vi "overwrite.vi"(0 "Enable":bool=TRUE, 4 "Overwrite":path=path "C:/Users/Clavius/Desktop/Database Query files/New_Database_Query.hdf5" caption="Overwrite path", 5 "error in (no error)":errorcluster) -> (14 "Save folder":path=path "C:/Users/Clavius/Desktop/Database Query files/New_Database_Query.hdf5" caption="File path", 17 "Cancelled?":bool, 18 "Overwrite exsisting file":bool, 19 "error out":errorcluster)   [LabVIEW 2012]
doc: "Displays a standard dialog box that prompts users to enter information, such as a user name and password.\n--------------------\n\nThis Express VI is configured as follows:\n\nMessage to Display to the User:A file with the name you have specificied already exsists. \nThe inputs are:"
panel:
  in  "OK2 2":bool caption="OK2"
  in  "New Save folder":path caption="Change Name:"
  out "String":string="A file with the name you have specificied already exsists. "
  in  "OK2":bool
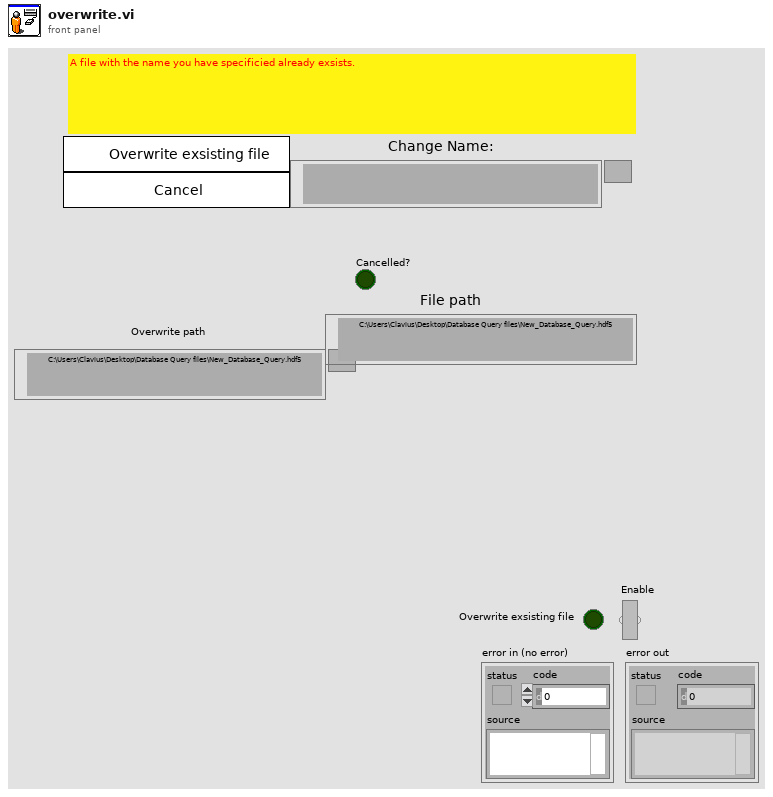
[diagram p1: front panel]
types:
  T1 = cluster{"Input Name":string, "Input Data Type":i32}[]
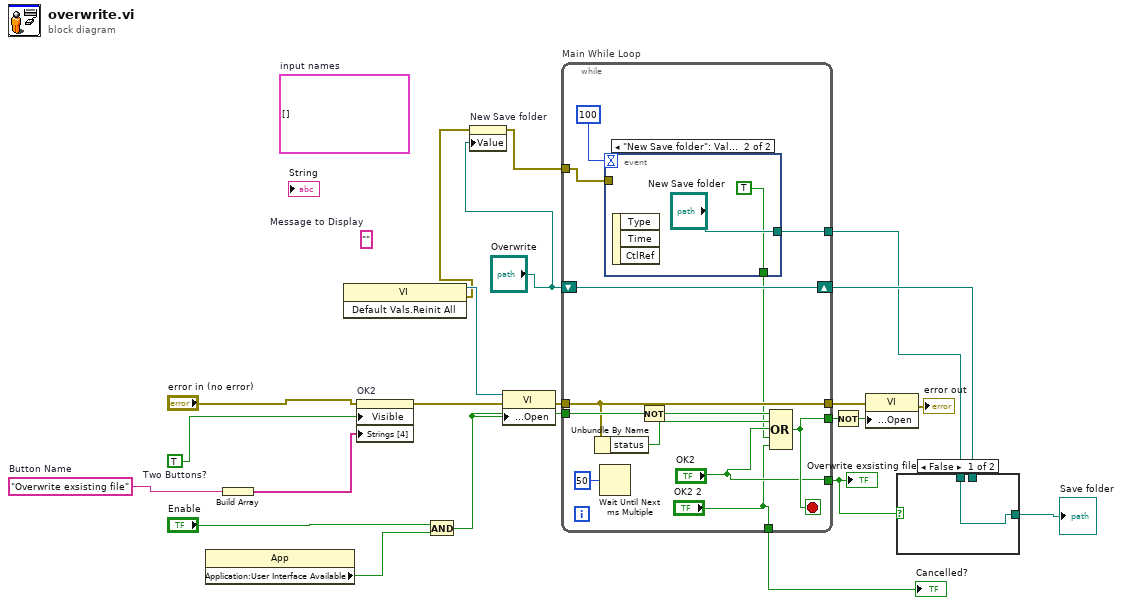
[diagram p0: block diagram]
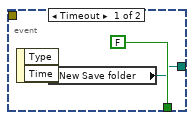
[diagram p3: hidden frame]
diagram:
  (unwired) T1 []  # input names
  w19 = "Overwrite exsisting file"  # Button Name
  (unwired) ""  # Message to Display
  w10 = TRUE  # Two Buttons?
  n1 = property class="App"() -> ("Application:User Interface Available"=w13:bool)  [unwired: 2 in, 2 out]
  n2 = Build Array(w19) -> (w20:string[])
  n3 = invoke class="VI" method="Default Vals.Reinit All"() -> (reference out=w12:refnum<vi>, error out=w1:errorcluster)  [unwired: 3 in, 1 out]
  n4 = property on="OK2" class="Bool"(error in="error in (no error)", "Visible"=w10, "Strings [4]"=w20) -> (error out=w9:errorcluster)  [unwired: 1 in, 1 out]
  n5 = And(x="Enable", y=w13) -> (x .and. y?=w14:bool)
  n6 = property on="New Save folder" class="Path"(error in=w1, "Value"="Overwrite") -> (error out=w2:errorcluster)  [unwired: 1 in, 1 out]
  n7 = property class="VI"(reference=w12, error in=w9, "Front Panel Window:Open"=w14) -> (error out=w18:errorcluster)  [unwired: 1 out]
  n8 = while "Main While Loop" {
    tunnel: ["OK2"] -> w8
    tunnel: w14 -> [w34]
    tunnel: [w32] -> w21
    tunnel: w18 -> [w31]
    tunnel: [w31] -> w17
    shift-right: [w28] -> w7
    shift-left: "Overwrite" -> [w28]
    tunnel: [w27] -> w5
    tunnel: ["OK2 2"] -> w4
    tunnel: w2 -> [w23]
    stop <- w32 stop-if-true
    n9 = Unbundle By Name(w31) -> ("status"=w30:bool)
    n10 = Wait Until Next ms Multiple(millisecond multiple=u32 50) -> ()  [unwired: 1 out]
    n11 = event shown="[1] \"New Save folder\": Value Change" {
      selector: _ -> [_ _]
      dyn-events: _ -> [_ _]
      timeout: 100 -> [_ _]
      tunnel: [w36 "New Save folder"] -> w27
      tunnel: [FALSE TRUE] -> w25
      tunnel: w23 -> [_ _]
      event Timeout {
        n12 = event-data() -> ()  [unwired: 1 in, 2 out]
        n13 = local read "New Save folder"() -> (w36:path)
      }
      event "New Save folder": Value Change {
        n14 = event-data() -> ()  [unwired: 1 in, 3 out]
      }
    }
    n15 = Not(x=w34) -> (.not. x?=w33:bool)
    n16 = Compound Arithmetic op=OR(w33, w30, "OK2", w25, "OK2 2") -> (w32:bool)
  }
  "Overwrite exsisting file" <- w8
  "Cancelled?" <- w4
  n17 = Not(x=w21) -> (.not. x?=w22:bool)
  n18 = property class="VI"(error in=w17, "Front Panel Window:Open"=w22) -> (error out=→"error out":errorcluster)  [unwired: 1 in, 1 out]
  n19 = case shown="False" w8 {
    tunnel: w7 -> [_ w41]
    tunnel: [w40 w41] -> w6
    tunnel: w5 -> [w40 _]
    frame False {
    }
    frame True {
    }
  }
  "Save folder" <- w6
